vi "Add Close Shutter.vi"(11 "Input Array":refnum<class "Message.lvclass">[](array[class])) -> (3 "Output Array":refnum<class "Message.lvclass">[](array[class]))   [LabVIEW 2018, in "Application.lvlib" / "Close Shutter Msg.lvclass"]
uses:
  Close Shutter Msg.lvclass
  <vilib>/ActorFramework/Message/Message.lvclass
  C:/Program Files/National Instruments/LabVIEW 2018/vi.lib/ActorFramework/Message/Message.lvclass
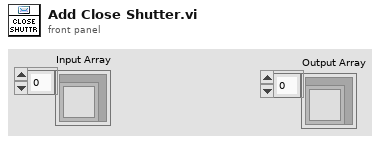
[diagram p1: front panel]
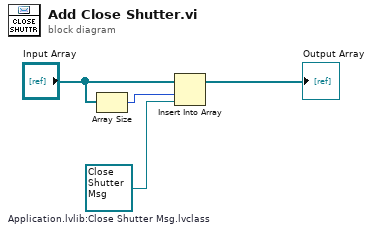
[diagram p0: block diagram]
diagram:
  w1 = refnum<class "Close Shutter Msg.lvclass"> refnum  # Application.lvlib:Close Shutter Msg.lvclass
  n1 = Array Size(array="Input Array") -> (size(s)=w2:i32)
  n2 = Insert Into Array(array="Input Array", index=w2, new element=w1) -> (→"Output Array":refnum<class "Message.lvclass">[])
